vi "Time Format String.vi"() -> ()   [LabVIEW 2013]
panel:
  out "appended path":path
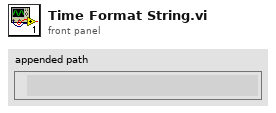
[diagram p1: front panel]
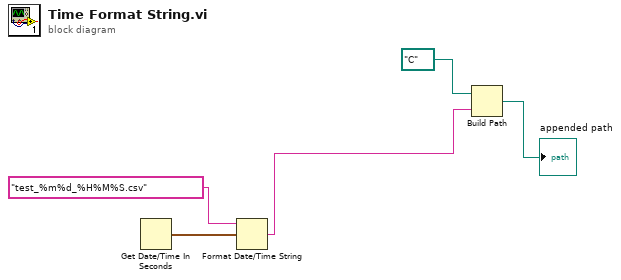
[diagram p0: block diagram]
diagram:
  n1 = Get Date/Time In Seconds() -> (seconds since 1Jan1904=w3:timestamp)
  n2 = Format Date/Time String(time format string (%c)="test_%m%d_%H%M%S.csv", seconds (now)=w3) -> (date/time string=w1:string)  [unwired: 1 in]
  n3 = Build Path(base path=path "C:/", name or relative path=w1) -> (appended path=→"appended path":path)
